vi "loopback cluster.vi"() -> ()   [LabVIEW 2013]
uses:
  Source/Pipes/Classes/Unix Pipe Reader/Open Pipe (reader).vi
  Source/Pipes/Classes/Unix Pipe Writer/Open Pipe (writer).vi
  Source/Pipes/Classes/Unix Pipe Reader/Close Pipe (reader).vi
  Source/Pipes/Classes/Unix Pipe Writer/Close Pipe (writer).vi
  <vilib>/NI/NI Linux RT Utilities/VIs/Public/Time/Get Clock Time (timespec).vi
  <vilib>/NI/NI Linux RT Utilities/Linux RT Utilities.lvlib
  Source/Pipes/Linux RT IPC.Pipes.lvlib
  Source/Pipes/Classes/Unix Pipe Writer/Unix Pipe Writer.lvclass
  Source/Pipes/Classes/Unix Pipe Reader/Unix Pipe Reader.lvclass
panel:
  out "read iterations":i32
  out "write iterations":i32
  in  "write":bool
  out "timed out":bool
  out "stop":bool
  out "pipe already exists?":bool
  in  "stop":bool
  out "time":cluster{"sec":u64, "nsec":u64}
  out "bytes read":i32
  out "error out":errorcluster
  out "bytes written":i32
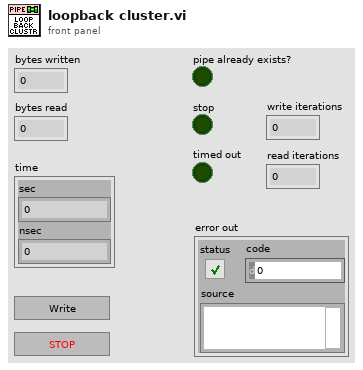
[diagram p1: front panel]
types:
  T1 = cluster{"Stop":bool, "Time":cluster{"sec":u64, "nsec":u64}}
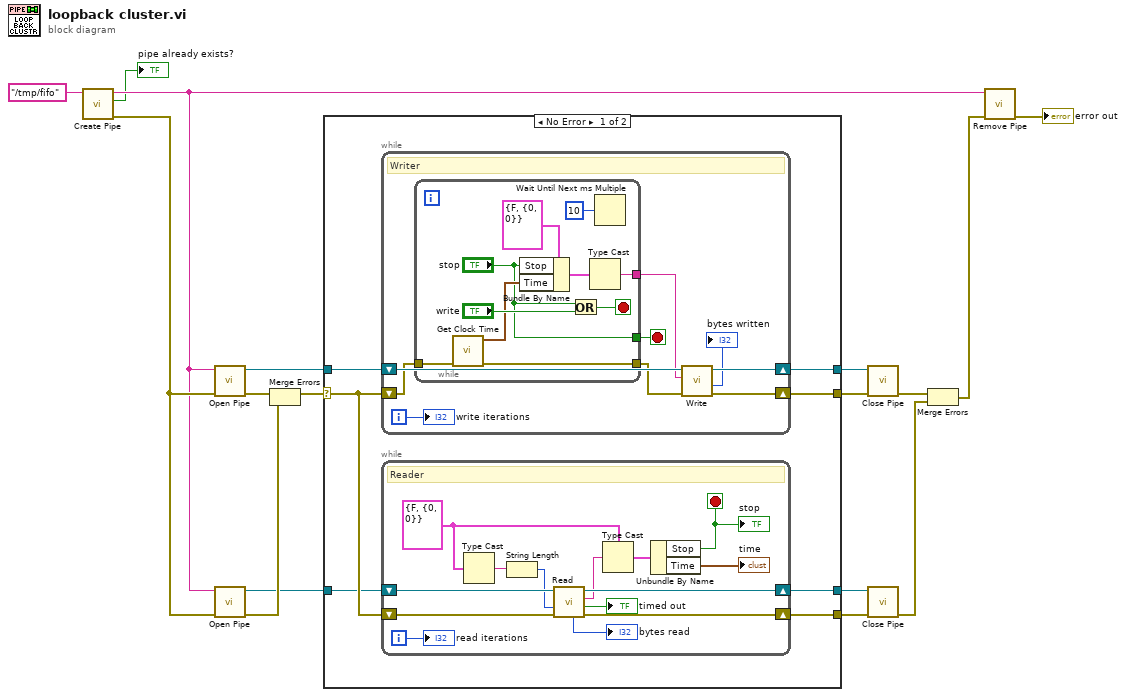
[diagram p0: block diagram]
diagram:
  n1 = call "Create Pipe.vi"("pathname in"="/tmp/fifo") -> ("error out"=w16:errorcluster, "pipe already exists?"=→"pipe already exists?":bool, "pathname out"=w15:string)  [unwired: 8 in]
  n2 = call-poly "Open Pipe.vi"("error in (no error)"=w16, "pathname in"=w15) -> ("error out"=w5:errorcluster, "pipe writer out"=w12:refnum<data-value>)  [unwired: 8 in]
  n3 = call-poly "Open Pipe.vi"("error in (no error)"=w16, "pathname in"=w15) -> ("error out"=w4:errorcluster, "pipe reader out"=w2:refnum<data-value>)  [unwired: 8 in]
  n4 = Merge Errors(w5, w4) -> (w3:errorcluster)
  n5 = case shown="No Error" w3 {
    selector: w3 -> [w19 w59]
    tunnel: w12 -> [w24 w60]
    tunnel: [w23 w60] -> w11
    tunnel: [w22 w59] -> w10
    tunnel: w2 -> [w18 w58]
    tunnel: [w21 w58] -> w9
    tunnel: [w20 w59] -> w8
    frame No Error {
      n6 = while {
        shift-right: [w47] -> w23
        shift-left: w24 -> [w44]
        shift-right: [w46] -> w22
        shift-left: w19 -> [w42]
        i -> [w45]
        stop <- w39 stop-if-true
        # "Writer"
        n7 = while {
          tunnel: [w53] -> w40
          tunnel: [w51] -> w41
          tunnel: w42 -> [w49]
          tunnel: ["stop"] -> w39
          stop <- w54 stop-if-true
          n8 = call-poly <vilib>:"Get Clock Time.vi"("error in (no error)"=w49) -> ("error out"=w51:errorcluster, "timespec"=w50:cluster{"sec":u64, "nsec":u64})  [unwired: 9 in]
          n9 = Bundle By Name(cluster=T1 {"Stop"=FALSE, "Time"={"sec"=0, "nsec"=0}}, "Stop"="stop", "Time"=w50) -> (w57:T1)
          n10 = Or(x="stop", y="write") -> (x .or. y?=w54:bool)
          n11 = Type Cast(x=w57) -> (*(type *) &x=w53:string)  [unwired: 1 in]
          n12 = Wait Until Next ms Multiple(millisecond multiple=u32 10 ("wait")) -> ()  [unwired: 1 out]
        }
        n13 = call "Write.vi"("error in (no error)"=w41, "data"=w40, "pipe writer in"=w44) -> ("error out"=w46:errorcluster, "bytes written"=→"bytes written":i32, "pipe writer out"=w47:refnum<data-value>)  [unwired: 6 in]
        "write iterations" <- w45
      }
      n14 = while {
        shift-right: [w33] -> w21
        shift-left: w18 -> [w37]
        shift-right: [w32] -> w20
        shift-left: w19 -> [w36]
        i -> [w25]
        stop <- w28 stop-if-true
        w34 = T1 {"Stop"=FALSE, "Time"={"sec"=0, "nsec"=0}}
        # "Reader"
        n15 = Type Cast(x=w34) -> (*(type *) &x=w38:string)  [unwired: 1 in]
        n16 = String Length(string=w38) -> (length=w35:i32)
        n17 = call "Read.vi"("error in (no error)"=w36, "bytes to read"=w35, "pipe reader in"=w37) -> ("error out"=w32:errorcluster, "timed out"=→"timed out":bool, "data"=w31:string, "pipe reader out"=w33:refnum<data-value>, "bytes read"=→"bytes read":i32)  [unwired: 4 in]
        n18 = Type Cast(type=w34, x=w31) -> (*(type *) &x=w30:T1)
        n19 = Unbundle By Name(w30) -> ("Stop"=w28:bool, "Time"=→"time":cluster{"sec":u64, "nsec":u64})
        "stop" <- w28
        "read iterations" <- w25
      }
    }
    frame Error {
    }
  }
  n20 = call-poly "Close Pipe.vi"("error in (no error)"=w10, "pipe in"=w11) -> ("error out"=w7:errorcluster)  [unwired: 8 in, 1 out]
  n21 = call-poly "Close Pipe.vi"("error in (no error)"=w8, "pipe in"=w9) -> ("error out"=w6:errorcluster)  [unwired: 8 in, 1 out]
  n22 = Merge Errors(w7, w6) -> (w1:errorcluster)
  n23 = call "Remove Pipe.vi"("error in (no error)"=w1, "pathname in"=w15) -> ("error out"=→"error out":errorcluster)  [unwired: 9 in]
